vi "SUB_COUNT_SPECIFIChar_fromString.vi"(1 "Find this char":string, 2 "Input String":string) -> (0 "Total Count":i32)   [LabVIEW 2011]
panel:
  out "Input  array":u8[](array[numeric])
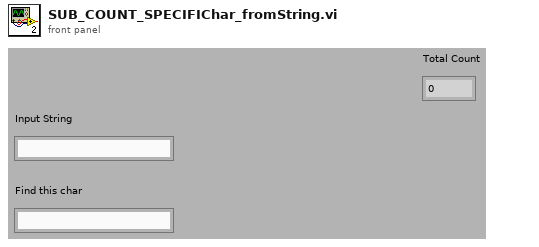
[diagram p1: front panel]
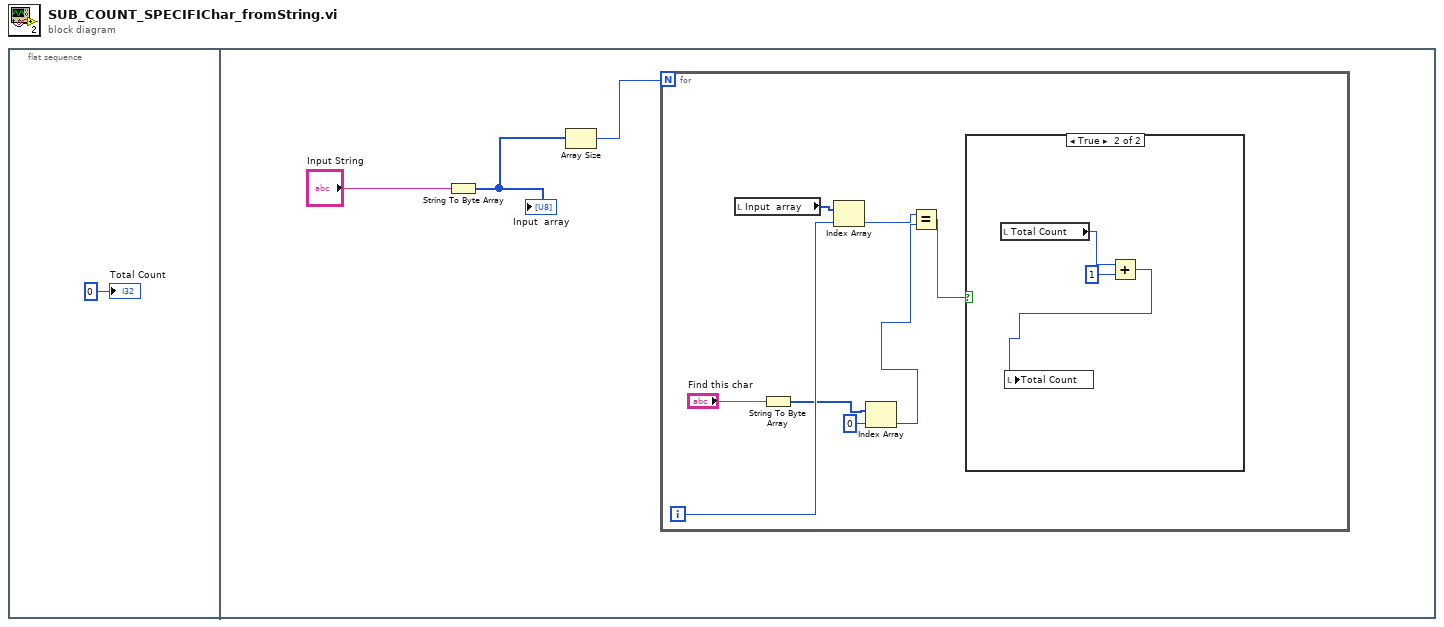
[diagram p0: block diagram]
diagram:
  n1 = flat-sequence {
    frame #0 {
      "Total Count" <- 0
    }
    frame #1 {
      n2 = String To Byte Array(string="Input String") -> (unsigned byte array=w3:u8[])
      "Input  array" <- w3
      n3 = Array Size(array=w3) -> (size(s)=w2:i32)
      n4 = for {
        N: w2 -> [_]
        i -> [w11]
        n5 = local read "Input  array"() -> (w12:u8[])
        n6 = String To Byte Array(string="Find this char") -> (unsigned byte array=w8:u8[])
        n7 = Index Array(array=w12, index=w11) -> (element=w10:u8)
        n8 = Index Array(array=w8, index=0) -> (element=w6:u8)
        n9 = Equal?(x=w10, y=w6) -> (x = y?=w5:bool)
        n10 = case shown="True" w5 {
          frame False {
          }
          frame True {
            n11 = local read "Total Count"() -> (w15:i32)
            n12 = Add(x=w15, y=1) -> (x+y=w13:i32)
            n13 = local write "Total Count"(w13) -> ()
          }
        }
      }
    }
  }
